vi "Lotis TII LS.vi"() -> ()   [LabVIEW 2015]
doc: "Example VI that demonstrates all library features."
uses:
  PL Lotis TII LS.lvclass
panel:
  in  "baud rate":u32(ring)=57600 items=["4800"=4800, "9600"=9600, "19200"=19200, "38400"=38400, "57600"=57600]
  in  "Tab Control":enum32{"Control", "Information"}(tab)
  in  "stop laser (keep lamp on)":bool
  in  "stop laser":bool
  in  "start laser":bool
  in  "configuration":T1={"device mode"=0, "error code"=0, "number of errors"=0, "cooling system"={"ready"=FALSE, "error"=FALSE}, "lamps"={"frequency, Hz"=0, "channel 1"={"trigger"=1, "state"=1, "energy, J"=0.0}, "channel 2"={"trigger"=1, "state"=1, "energy, J"=0.0}, "amplifier"={"enabled"=FALSE}, "off delay, s"=0, "number of shots"=0, "operation time, min."=0}, "Q-switches"={"frequency, Hz"=0.0, "trigger"=1, "channel 1"={"on"=FALSE, "delay, ns"=0}, "channel 2"={"on"=FALSE, "delay, ns"=0}, "number of shots"=0}, "shutters"={"channel 1"={"open"=FALSE}, "channel 1"={"open"=FALSE}}, "external device state index"=0, "external device flags"=[], "radiation energy, mJ"={"channel 1"=0, "channel 2"=0}, "lamp to Q-switch frequency ratio"=0, "4th harmonic crystal T, °C"=0.0} {"Q-switches"."trigger" items=["always on", "internal", "external (primary)", "external (secondary)", "single shot"]; "lamps"."channel 2"."state" items=["off"=0, "on"=1, "pulses"=3]; "lamps"."channel 2"."trigger" items=["internal"=1, "external"=2, "single shot"=3]; "lamps"."channel 1"."state" items=["off"=0, "on"=1, "pulses"=3]; "lamps"."channel 1"."trigger" items=["internal"=1, "external"=2, "single shot"=3]; "device mode" items=["independent", "primary", "secondary"]}
  in  "reset errors":bool
  out "device name":string
  out "serial number":string
  out "device information":T2 {"optical channels" items=["no", "single", "double", "double with ns delays"]; "cooling system" items=["no", "single", "double", "internal"]; "laser system" items=["single lamp", "double lamp", "long pulse", "double lamp PICO", "single lamp with delay", "extended synchronization"]}
  out "external device states":u8[](array[numeric]) format="%x"
  out "message table index":u8
  out "power supply information":T3
  out "service information":T4
  in  "default":bool
  in  "restore":bool
  in  "save":bool
  in  "port":refnum<visa-resource-name>
  out "error":errorcluster
  in  "stop":bool
  out "Lotis":refnum<class "PL Lotis TII LS.lvclass">
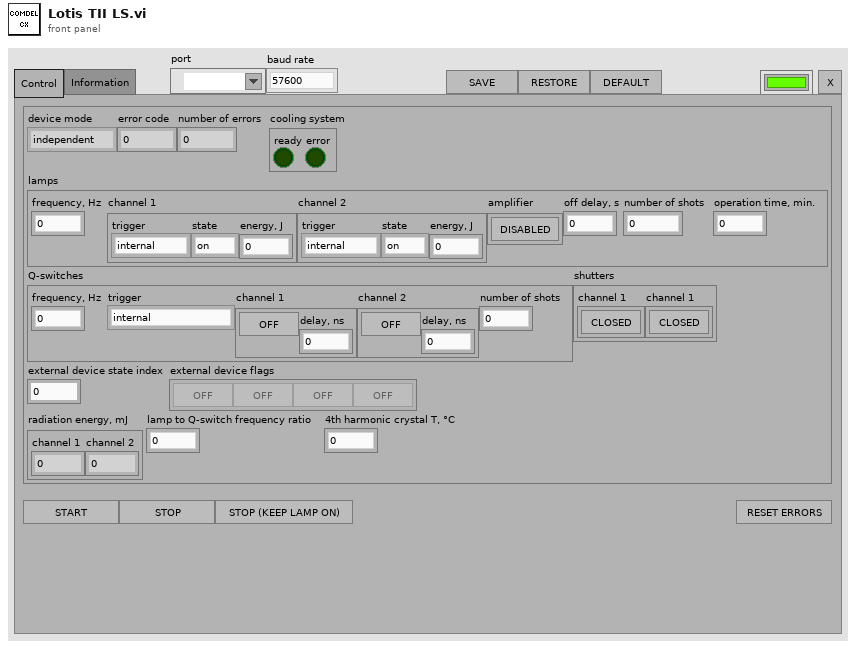
[diagram p1: front panel]
types:
  T1 = cluster{"device mode":u16, "error code":u8, "number of errors":u8, "cooling system":cluster{"ready":bool, "error":bool}, "lamps":cluster{"frequency, Hz":u32, "channel 1":cluster{"trigger":u16, "state":u16, "energy, J":dbl}, "channel 2":cluster{"trigger":u16, "state":u16, "energy, J":dbl}, "amplifier":cluster{"enabled":bool}, "off delay, s":u32, "number of shots":u32, "operation time, min.":u32}, "Q-switches":cluster{"frequency, Hz":dbl, "trigger":u16, "channel 1":cluster{"on":bool, "delay, ns":u32}, "channel 2":cluster{"on":bool, "delay, ns":u32}, "number of shots":u32}, "shutters":cluster{"channel 1":cluster{"open":bool}, "channel 1":cluster{"open":bool}}, "external device state index":u8, "external device flags":bool[], "radiation energy, mJ":cluster{"channel 1":u32, "channel 2":u32}, "lamp to Q-switch frequency ratio":u32, "4th harmonic crystal T, °C":dbl}
  T2 = cluster{"model id":u16, "laser name":string, "laser system":u16, "optical channels":u16, "number of radiation indicators":u16, "cooling system":u16, "control buttons":bool, "external door interlock":bool, "external interlock 1":bool, "external interlock 2":bool, "external lamp control":bool, "saving lamp energy":bool, "variable frequency":bool, "extended frequency range":bool, "FH oven temperature":bool, "external device register":u8, "exernal device flags":bool[], "4th harmonic crystal Tmax, °C":u32, "lamps":cluster{"frequency, Hz":cluster{"min":u32, "max":u32, "default":u32}, "channel 1":cluster{"Emin, J":u32, "Emax, J":u32, "Edefault, J":u32}, "channel 2":cluster{"Emin, J":u32, "Emax, J":u32, "Edefault, J":u32}}, "radiation":cluster{"channel 1":cluster{"Emax, mJ":u32}, "channel 2":cluster{"Emax, mJ":u32}}, "Q-switches":cluster{"channel 1":cluster{"delay step, ns":u32}, "channel 2":cluster{"delay step, ns":u32}}}
  T3 = cluster{"channel 1":cluster{"capacitance, uF":u32, "Urequired, V":u32, "Umeasured, V":u32, "Umin, V":u32, "Umax, V":u32}, "channel 2":cluster{"capacitance, uF":u32, "Urequired, V":u32, "Umeasured, V":u32, "Umin, V":u32, "Umax, V":u32}, "Ucorrection-, V":u32, "Ucorrection+, V":u32, "Udeviation max, %":u32}
  T4 = cluster{"lamp energy averaging":u32, "radiation energy averaging":u32, "lamp shots max":u32, "lamp operaition time  max, min.":u32, "lamp external period min, ms":u32, "lamp external period max, ms":u32}
  T5 = cluster{"device mode":u16, "error code":u8, "number of errors":u8, "cooling system":cluster{"ready":bool, "error":bool}, "lamps":cluster{"frequency, Hz":u32, "channel 1":cluster{"trigger":u16, "state":u16, "energy, J":dbl}, "channel 2":cluster{"trigger":u16, "state":u16, "energy, J":dbl}, "amplifier":cluster{"enabled":bool}, "off delay, s":u32, "number of shots":u32, "operation time, min.":u32}, "Q-switches":cluster{"frequency, Hz":dbl, "trigger":u16, "channel 1":cluster{"on":bool, "delay, ns":u32}, "channel 2":cluster{"on":bool, "delay ,ns":u32}, "number of shots":u32}, "shutters":cluster{"channel 1":cluster{"open":bool}, "channel 2":cluster{"open":bool}}, "external device state index":u8, "exernal device flags":bool[], "radiation energy, mJ":cluster{"channel 1":u32, "channel 2":u32}, "lamp to Q-switch frequency ratio":u32, "4th harmonic crystal T, °C":dbl}
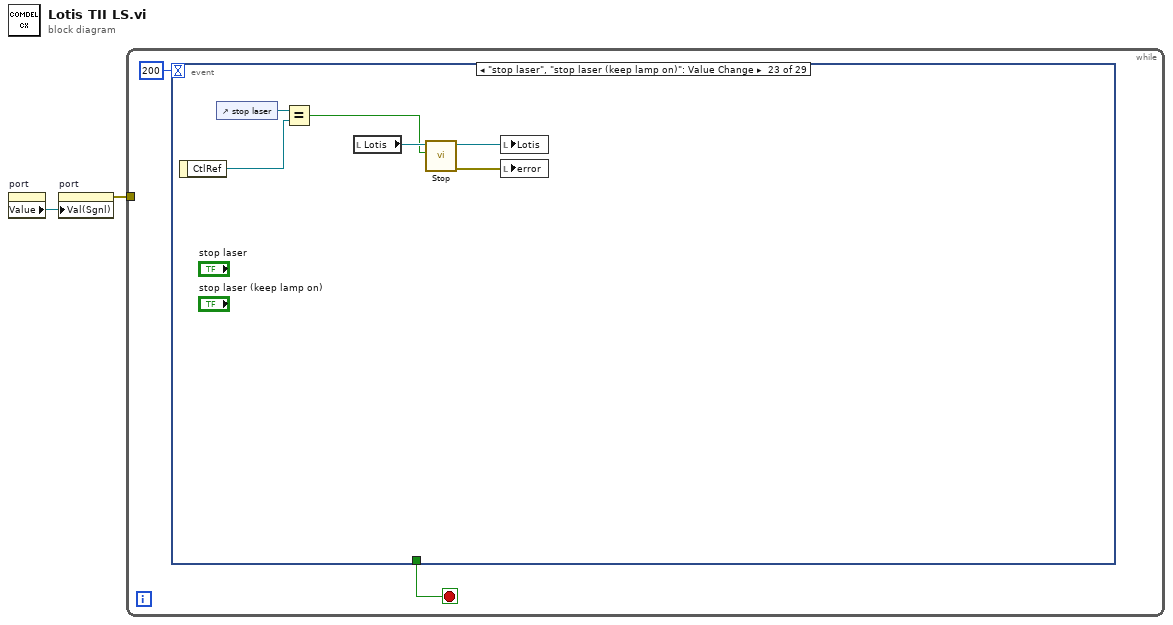
[diagram p0: block diagram]
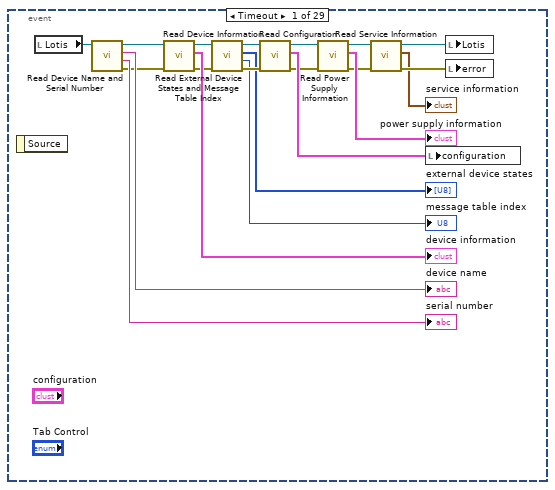
[diagram p2: hidden frame]
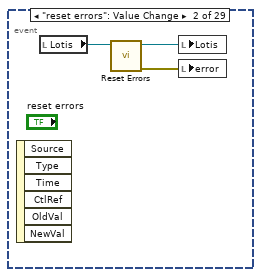
[diagram p3: hidden frame]
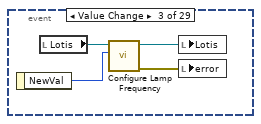
[diagram p4: hidden frame]
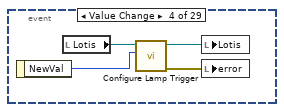
[diagram p5: hidden frame]
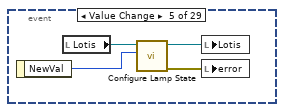
[diagram p6: hidden frame]
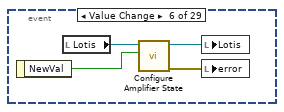
[diagram p7: hidden frame]
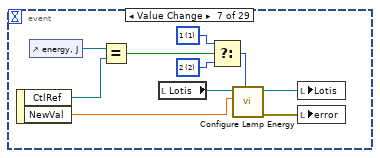
[diagram p8: hidden frame]
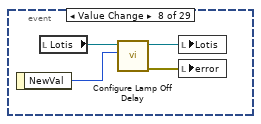
[diagram p9: hidden frame]
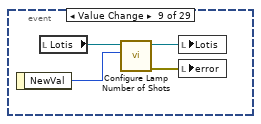
[diagram p10: hidden frame]
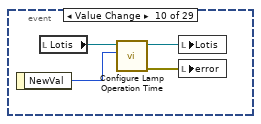
[diagram p11: hidden frame]
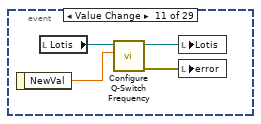
[diagram p12: hidden frame]
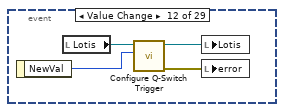
[diagram p13: hidden frame]
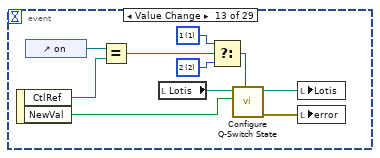
[diagram p14: hidden frame]
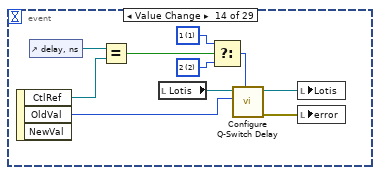
[diagram p15: hidden frame]
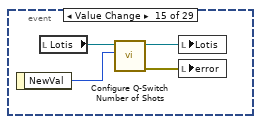
[diagram p16: hidden frame]
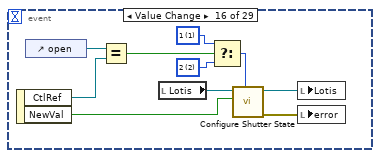
[diagram p17: hidden frame]
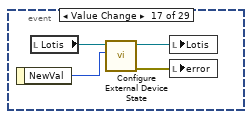
[diagram p18: hidden frame]
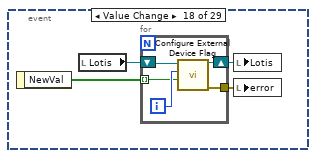
[diagram p19: hidden frame]
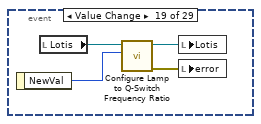
[diagram p20: hidden frame]
diagram:
  n1 = property on="port" class="VISAName"() -> ("Value"=w1:refnum<visa-resource-name>)  [unwired: 2 in, 2 out]
  n2 = property on="port" class="VISAName"("Val(Sgnl)"=w1) -> (error out=w2:errorcluster)  [unwired: 2 in, 1 out]
  n3 = while {
    tunnel: w2 -> [_]
    stop <- w3 stop-if-true
    n4 = event shown="[22] \"stop laser\", \"stop laser (keep lamp on)\": Value Change" {
      selector: _ -> [_ _ _ _ _ _ _ _ _ _ _ _ _ _ _ _ _ _ _ _ _ _ _ _ _ _ _ _ _]
      dyn-events: _ -> [_ _ _ _ _ _ _ _ _ _ _ _ _ _ _ _ _ _ _ _ _ _ _ _ _ _ _ _ _]
      timeout: 200 -> [_ _ _ _ _ _ _ _ _ _ _ _ _ _ _ _ _ _ _ _ _ _ _ _ _ _ _ _ _]
      tunnel: [_ _ _ _ _ _ _ _ _ _ _ _ _ _ _ _ _ _ _ _ _ _ _ _ _ _ _ _ TRUE ("stop")] -> w3
      event Timeout {
        n5 = event-data() -> ()  [unwired: 1 in, 1 out]
        n6 = local read "Lotis"() -> (w25:refnum<class "PL Lotis TII LS.lvclass">)
        n7 = call "Read Device Name and Serial Number.vi"("Lotis in"=w25) -> ("error out"=w21:errorcluster, "serial number"=→"serial number":string, "name"=→"device name":string, "Lotis out"=w22:refnum<class "PL Lotis TII LS.lvclass">)  [unwired: 7 in]
        n8 = call "Read Device Information.vi"("error in (no error)"=w21, "Lotis in"=w22) -> ("error out"=w18:errorcluster, "information"=→"device information":T2, "Lotis out"=w19:refnum<class "PL Lotis TII LS.lvclass">)  [unwired: 7 in]
        n9 = call "Read External Device States and Message Table Index.vi"("error in (no error)"=w18, "Lotis in"=w19) -> ("error out"=w17:errorcluster, "message table index"=→"message table index":u8, "external device states"=→"external device states":u8[], "Lotis out"=w16:refnum<class "PL Lotis TII LS.lvclass">)  [unwired: 6 in]
        n10 = call "Read Configuration.vi"("error in (no error)"=w17, "Lotis in"=w16) -> ("error out"=w11:errorcluster, "configuration"=w13:T5, "Lotis out"=w12:refnum<class "PL Lotis TII LS.lvclass">)  [unwired: 7 in]
        n11 = call "Read Power Supply Information.vi"("error in (no error)"=w11, "Lotis in"=w12) -> ("error out"=w8:errorcluster, "information"=→"power supply information":T3, "Lotis out"=w9:refnum<class "PL Lotis TII LS.lvclass">)  [unwired: 7 in]
        n12 = call "Read Service Information.vi"("error in (no error)"=w8, "Lotis in"=w9) -> ("error out"=w7:errorcluster, "information"=→"service information":T4, "Lotis out"=w6:refnum<class "PL Lotis TII LS.lvclass">)  [unwired: 7 in]
        n13 = local write "configuration"(w13) -> ()
        n14 = local write "Lotis"(w6) -> ()
        n15 = local write "error"(w7) -> ()
      }
      event "reset errors": Value Change {
        n16 = event-data() -> ()  [unwired: 1 in, 6 out]
        n17 = local read "Lotis"() -> (w28:refnum<class "PL Lotis TII LS.lvclass">)
        n18 = call "Reset Errors.vi"("Lotis in"=w28) -> ("error out"=w26:errorcluster, "Lotis out"=w27:refnum<class "PL Lotis TII LS.lvclass">)  [unwired: 9 in]
        n19 = local write "Lotis"(w27) -> ()
        n20 = local write "error"(w26) -> ()
      }
      event "configuration.lamps.frequency, Hz": Value Change {
        n21 = event-data() -> ("NewVal"=w29:u32)  [unwired: 1 in]
        n22 = local read "Lotis"() -> (w30:refnum<class "PL Lotis TII LS.lvclass">)
        n23 = call "Configure Lamp Frequency.vi"("frequency, Hz"=w29, "Lotis in"=w30) -> ("error out"=w31:errorcluster, "Lotis out"=w32:refnum<class "PL Lotis TII LS.lvclass">)  [unwired: 8 in]
        n24 = local write "Lotis"(w32) -> ()
        n25 = local write "error"(w31) -> ()
      }
      event "configuration.lamps.channel 1.trigger": Value Change {
        n26 = event-data() -> ("NewVal"=w33:u16)  [unwired: 1 in]
        n27 = local read "Lotis"() -> (w36:refnum<class "PL Lotis TII LS.lvclass">)
        n28 = call "Configure Lamp Trigger.vi"("trigger"=w33, "Lotis in"=w36) -> ("error out"=w34:errorcluster, "Lotis out"=w35:refnum<class "PL Lotis TII LS.lvclass">)  [unwired: 8 in]
        n29 = local write "Lotis"(w35) -> ()
        n30 = local write "error"(w34) -> ()
      }
      event "configuration.lamps.channel 1.state": Value Change {
        n31 = event-data() -> ("NewVal"=w38:u16)  [unwired: 1 in]
        n32 = local read "Lotis"() -> (w37:refnum<class "PL Lotis TII LS.lvclass">)
        n33 = call "Configure Lamp State.vi"("state"=w38, "Lotis in"=w37) -> ("error out"=w39:errorcluster, "Lotis out"=w40:refnum<class "PL Lotis TII LS.lvclass">)  [unwired: 8 in]
        n34 = local write "Lotis"(w40) -> ()
        n35 = local write "error"(w39) -> ()
      }
      event "configuration.lamps.amplifier.enabled": Value Change {
        n36 = event-data() -> ("NewVal"=w41:bool)  [unwired: 1 in]
        n37 = local read "Lotis"() -> (w44:refnum<class "PL Lotis TII LS.lvclass">)
        n38 = call "Configure Amplifier State.vi"("lamp enabled"=w41, "Lotis in"=w44) -> ("error out"=w42:errorcluster, "Lotis out"=w43:refnum<class "PL Lotis TII LS.lvclass">)  [unwired: 8 in]
        n39 = local write "Lotis"(w43) -> ()
        n40 = local write "error"(w42) -> ()
      }
      event "configuration.lamps.channel 1.energy, J", "configuration.lamps.channel 2.energy, J": Value Change {
        w52 = u16 2 items=["1"=1, "2"=2]
        w51 = u16 1 items=["1"=1, "2"=2]
        n41 = event-data() -> ("CtlRef"=w45:refnum<vi>, "NewVal"=w46:dbl)  [unwired: 1 in]
        n42 = control-ref of="energy, J"() -> (w54:refnum<vi>)
        n43 = Equal?(x=w54, y=w45) -> (x = y?=w53:bool)
        n44 = local read "Lotis"() -> (w50:refnum<class "PL Lotis TII LS.lvclass">)
        n45 = Select(t=w51, s=w53, f=w52) -> (s? t:f=w49:u16)
        n46 = call "Configure Lamp Energy.vi"("channel (1)"=w49, "energy, J"=w46, "Lotis in"=w50) -> ("error out"=w47:errorcluster, "Lotis out"=w48:refnum<class "PL Lotis TII LS.lvclass">)  [unwired: 7 in]
        n47 = local write "Lotis"(w48) -> ()
        n48 = local write "error"(w47) -> ()
      }
      event "configuration.lamps.off delay, s": Value Change {
        n49 = event-data() -> ("NewVal"=w56:u32)  [unwired: 1 in]
        n50 = local read "Lotis"() -> (w55:refnum<class "PL Lotis TII LS.lvclass">)
        n51 = call "Configure Lamp Off Delay.vi"("off delay, s"=w56, "Lotis in"=w55) -> ("error out"=w57:errorcluster, "Lotis out"=w58:refnum<class "PL Lotis TII LS.lvclass">)  [unwired: 8 in]
        n52 = local write "Lotis"(w58) -> ()
        n53 = local write "error"(w57) -> ()
      }
      event "configuration.lamps.number of shots": Value Change {
        n54 = event-data() -> ("NewVal"=w59:u32)  [unwired: 1 in]
        n55 = local read "Lotis"() -> (w60:refnum<class "PL Lotis TII LS.lvclass">)
        n56 = call "Configure Lamp Number of Shots.vi"("number of shots"=w59, "Lotis in"=w60) -> ("error out"=w61:errorcluster, "Lotis out"=w62:refnum<class "PL Lotis TII LS.lvclass">)  [unwired: 8 in]
        n57 = local write "Lotis"(w62) -> ()
        n58 = local write "error"(w61) -> ()
      }
      event "configuration.lamps.operation time, min.": Value Change {
        n59 = event-data() -> ("NewVal"=w63:u32)  [unwired: 1 in]
        n60 = local read "Lotis"() -> (w65:refnum<class "PL Lotis TII LS.lvclass">)
        n61 = call "Configure Lamp Operation Time.vi"("operation time, min."=w63, "Lotis in"=w65) -> ("error out"=w64:errorcluster, "Lotis out"=w66:refnum<class "PL Lotis TII LS.lvclass">)  [unwired: 8 in]
        n62 = local write "Lotis"(w66) -> ()
        n63 = local write "error"(w64) -> ()
      }
      event "configuration.Q-switches.frequency, Hz": Value Change {
        n64 = event-data() -> ("NewVal"=w67:dbl)  [unwired: 1 in]
        n65 = local read "Lotis"() -> (w68:refnum<class "PL Lotis TII LS.lvclass">)
        n66 = call "Configure Q-Switch Frequency.vi"("frequency, Hz"=w67, "Lotis in"=w68) -> ("error out"=w69:errorcluster, "Lotis out"=w70:refnum<class "PL Lotis TII LS.lvclass">)  [unwired: 8 in]
        n67 = local write "Lotis"(w70) -> ()
        n68 = local write "error"(w69) -> ()
      }
      event "configuration.Q-switches.trigger": Value Change {
        n69 = event-data() -> ("NewVal"=w72:u16)  [unwired: 1 in]
        n70 = local read "Lotis"() -> (w71:refnum<class "PL Lotis TII LS.lvclass">)
        n71 = call "Configure Q-Switch Trigger.vi"("trigger"=w72, "Lotis in"=w71) -> ("error out"=w73:errorcluster, "Lotis out"=w74:refnum<class "PL Lotis TII LS.lvclass">)  [unwired: 8 in]
        n72 = local write "Lotis"(w74) -> ()
        n73 = local write "error"(w73) -> ()
      }
      event "configuration.Q-switches.channel 1.on", "configuration.Q-switches.channel 2.on": Value Change {
        w77 = u16 2 items=["1"=1, "2"=2]
        w75 = u16 1 items=["1"=1, "2"=2]
        n74 = event-data() -> ("CtlRef"=w79:refnum<vi>, "NewVal"=w81:bool)  [unwired: 1 in]
        n75 = control-ref of="on"() -> (w80:refnum<vi>)
        n76 = Equal?(x=w80, y=w79) -> (x = y?=w78:bool)
        n77 = local read "Lotis"() -> (w82:refnum<class "PL Lotis TII LS.lvclass">)
        n78 = Select(t=w75, s=w78, f=w77) -> (s? t:f=w76:u16)
        n79 = call "Configure Q-Switch State.vi"("channel (1)"=w76, "on"=w81, "Lotis in"=w82) -> ("error out"=w83:errorcluster, "Lotis out"=w84:refnum<class "PL Lotis TII LS.lvclass">)  [unwired: 7 in]
        n80 = local write "Lotis"(w84) -> ()
        n81 = local write "error"(w83) -> ()
      }
      event "configuration.Q-switches.channel 1.delay, ns", "configuration.Q-switches.channel 2.delay, ns": Value Change {
        w91 = u16 2 items=["1"=1, "2"=2]
        w90 = u16 1 items=["1"=1, "2"=2]
        n82 = event-data() -> ("CtlRef"=w93:refnum<vi>, "OldVal"=w86:u32)  [unwired: 1 in, 1 out]
        n83 = control-ref of="delay, ns"() -> (w94:refnum<vi>)
        n84 = Equal?(x=w94, y=w93) -> (x = y?=w92:bool)
        n85 = local read "Lotis"() -> (w87:refnum<class "PL Lotis TII LS.lvclass">)
        n86 = Select(t=w90, s=w92, f=w91) -> (s? t:f=w88:u16)
        n87 = call "Configure Q-Switch Delay.vi"("channel (1)"=w88, "delay, ns"=w86, "Lotis in"=w87) -> ("error out"=w85:errorcluster, "Lotis out"=w89:refnum<class "PL Lotis TII LS.lvclass">)  [unwired: 7 in]
        n88 = local write "Lotis"(w89) -> ()
        n89 = local write "error"(w85) -> ()
      }
      event "configuration.Q-switches.number of shots": Value Change {
        n90 = event-data() -> ("NewVal"=w95:u32)  [unwired: 1 in]
        n91 = local read "Lotis"() -> (w98:refnum<class "PL Lotis TII LS.lvclass">)
        n92 = call "Configure Q-Switch Number of Shots.vi"("number of shots"=w95, "Lotis in"=w98) -> ("error out"=w96:errorcluster, "Lotis out"=w97:refnum<class "PL Lotis TII LS.lvclass">)  [unwired: 8 in]
        n93 = local write "Lotis"(w97) -> ()
        n94 = local write "error"(w96) -> ()
      }
      event "configuration.shutters.channel 1.open", "configuration.shutters.channel 1.open": Value Change {
        w105 = u16 2 items=["1"=1, "2"=2]
        w104 = u16 1 items=["1"=1, "2"=2]
        n95 = event-data() -> ("CtlRef"=w107:refnum<vi>, "NewVal"=w100:bool)  [unwired: 1 in]
        n96 = control-ref of="open"() -> (w108:refnum<vi>)
        n97 = Equal?(x=w108, y=w107) -> (x = y?=w106:bool)
        n98 = local read "Lotis"() -> (w101:refnum<class "PL Lotis TII LS.lvclass">)
        n99 = Select(t=w104, s=w106, f=w105) -> (s? t:f=w102:u16)
        n100 = call "Configure Shutter State.vi"("channel (1)"=w102, "open"=w100, "Lotis in"=w101) -> ("error out"=w99:errorcluster, "Lotis out"=w103:refnum<class "PL Lotis TII LS.lvclass">)  [unwired: 7 in]
        n101 = local write "Lotis"(w103) -> ()
        n102 = local write "error"(w99) -> ()
      }
      event "configuration.external device state index": Value Change {
        n103 = event-data() -> ("NewVal"=w109:u8)  [unwired: 1 in]
        n104 = local read "Lotis"() -> (w112:refnum<class "PL Lotis TII LS.lvclass">)
        n105 = call "Configure External Device State.vi"("state index"=w109, "Lotis in"=w112) -> ("error out"=w110:errorcluster, "Lotis out"=w111:refnum<class "PL Lotis TII LS.lvclass">)  [unwired: 8 in]
        n106 = local write "Lotis"(w111) -> ()
        n107 = local write "error"(w110) -> ()
      }
      event "configuration.external device flags": Value Change {
        n108 = event-data() -> ("NewVal"=w113:bool[])  [unwired: 1 in]
        n109 = local read "Lotis"() -> (w116:refnum<class "PL Lotis TII LS.lvclass">)
        n110 = for {
          tunnel: [w119] -> w114
          shift-right: [w120] -> w115
          shift-left: w116 -> [w121]
          tunnel: w113 -> [w117] mode=indexing
          i -> [w118]
          n111 = call "Configure External Device Flag.vi"("on"=w117, "flag index"=w118, "Lotis in"=w121) -> ("error out"=w119:errorcluster, "Lotis out"=w120:refnum<class "PL Lotis TII LS.lvclass">)  [unwired: 7 in]
        }
        n112 = local write "Lotis"(w115) -> ()
        n113 = local write "error"(w114) -> ()
      }
      event "configuration.lamp to Q-switch frequency ratio": Value Change {
        n114 = event-data() -> ("NewVal"=w122:u32)  [unwired: 1 in]
        n115 = local read "Lotis"() -> (w123:refnum<class "PL Lotis TII LS.lvclass">)
        n116 = call "Configure Lamp to Q-Switch Frequency Ratio.vi"("ratio"=w122, "Lotis in"=w123) -> ("error out"=w124:errorcluster, "Lotis out"=w125:refnum<class "PL Lotis TII LS.lvclass">)  [unwired: 8 in]
        n117 = local write "Lotis"(w125) -> ()
        n118 = local write "error"(w124) -> ()
      }
      event "configuration.4th harmonic crystal T, °C": Value Change {
        n119 = event-data() -> ("NewVal"=w126:dbl)  [unwired: 1 in]
        n120 = local read "Lotis"() -> (w127:refnum<class "PL Lotis TII LS.lvclass">)
        n121 = call "Configure 4th Harmonic Crystal Temperature.vi"("T, °C"=w126, "Lotis in"=w127) -> ("error out"=w128:errorcluster, "Lotis out"=w129:refnum<class "PL Lotis TII LS.lvclass">)  [unwired: 8 in]
        n122 = local write "Lotis"(w129) -> ()
        n123 = local write "error"(w128) -> ()
      }
      event "save": Value Change {
        n124 = event-data() -> ()  [unwired: 1 in, 1 out]
        n125 = local read "Lotis"() -> (w132:refnum<class "PL Lotis TII LS.lvclass">)
        n126 = call "Save Configuration.vi"("Lotis in"=w132) -> ("error out"=w130:errorcluster, "Lotis out"=w131:refnum<class "PL Lotis TII LS.lvclass">)  [unwired: 9 in]
        n127 = local write "Lotis"(w131) -> ()
        n128 = local write "error"(w130) -> ()
      }
      event "start laser": Value Change {
        n129 = event-data() -> ()  [unwired: 1 in, 1 out]
        n130 = local read "Lotis"() -> (w133:refnum<class "PL Lotis TII LS.lvclass">)
        n131 = call "Start.vi"("Lotis in"=w133) -> ("error out"=w134:errorcluster, "Lotis out"=w135:refnum<class "PL Lotis TII LS.lvclass">)  [unwired: 9 in]
        n132 = local write "Lotis"(w135) -> ()
        n133 = local write "error"(w134) -> ()
      }
      event "stop laser", "stop laser (keep lamp on)": Value Change {
        n134 = event-data() -> ("CtlRef"=w137:refnum<vi>)  [unwired: 1 in]
        n135 = control-ref of="stop laser"() -> (w138:refnum<vi>)
        n136 = Equal?(x=w138, y=w137) -> (x = y?=w136:bool)
        n137 = local read "Lotis"() -> (w139:refnum<class "PL Lotis TII LS.lvclass">)
        n138 = call "Stop.vi"("switch lamp off (true)"=w136, "Lotis in"=w139) -> ("error out"=w140:errorcluster, "Lotis out"=w141:refnum<class "PL Lotis TII LS.lvclass">)  [unwired: 8 in]
        n139 = local write "Lotis"(w141) -> ()
        n140 = local write "error"(w140) -> ()
      }
      event "restore": Value Change {
        n141 = event-data() -> ()  [unwired: 1 in, 1 out]
        n142 = local read "Lotis"() -> (w142:refnum<class "PL Lotis TII LS.lvclass">)
        n143 = call "Restore Configuration.vi"("Lotis in"=w142) -> ("error out"=w143:errorcluster, "Lotis out"=w144:refnum<class "PL Lotis TII LS.lvclass">)  [unwired: 9 in]
        n144 = local write "Lotis"(w144) -> ()
        n145 = local write "error"(w143) -> ()
      }
      event "default": Value Change {
        n146 = event-data() -> ()  [unwired: 1 in, 1 out]
        n147 = local read "Lotis"() -> (w145:refnum<class "PL Lotis TII LS.lvclass">)
        n148 = call "Restore Default Configuration.vi"("Lotis in"=w145) -> ("error out"=w146:errorcluster, "Lotis out"=w147:refnum<class "PL Lotis TII LS.lvclass">)  [unwired: 9 in]
        n149 = local write "Lotis"(w147) -> ()
        n150 = local write "error"(w146) -> ()
      }
      event "port": Value Change {
        n151 = event-data() -> ()  [unwired: 1 in, 6 out]
        n152 = local read "Lotis"() -> (w154:refnum<class "PL Lotis TII LS.lvclass">)
        n153 = call "Close.vi"("Comdel in"=w154) -> ("error out"=w149:errorcluster)  [unwired: 10 in]
        n154 = call <vilib>:"Clear Errors.vi"("error in (no error)"=w149) -> ("error out"=w151:errorcluster)  [unwired: 5 in, 1 out]
        n155 = local read "baud rate"() -> (w148:u32)
        n156 = call "Initialize.vi"("error in (no error)"=w151, "baud rate (57600)"=w148, "port"="port") -> ("error out"=→"error":errorcluster, "Lotis out"=→"Lotis":refnum<class "PL Lotis TII LS.lvclass">)  [unwired: 7 in]
      }
      event "baud rate": Value Change {
        n157 = event-data() -> ("NewVal"=w156:u32)  [unwired: 1 in]
        n158 = local read "Lotis"() -> (w157:refnum<class "PL Lotis TII LS.lvclass">)
        n159 = property on="port" class="VISAName"() -> ("Value"=w155:refnum<visa-resource-name>)  [unwired: 2 in, 2 out]
        n160 = call "Configure Baud Rate.vi"("baud rate"=w156, "Lotis in"=w157) -> ("error out"=w158:errorcluster, "Lotis out"=w159:refnum<class "PL Lotis TII LS.lvclass">)  [unwired: 8 in]
        n161 = property on="port" class="VISAName"("Val(Sgnl)"=w155) -> ()  [unwired: 2 in, 2 out]
        n162 = local write "Lotis"(w159) -> ()
        n163 = local write "error"(w158) -> ()
      }
      event "error": Mouse Up {
        n164 = event-data() -> ()  [unwired: 1 in, 1 out]
        n165 = local read "error"() -> (w160:errorcluster)
        n166 = call <vilib>:"Simple Error Handler.vi"("error in (no error)"=w160) -> ()  [unwired: 4 in, 5 out]
      }
      event "stop": Value Change {
        n167 = event-data() -> ()  [unwired: 1 in, 1 out]
        n168 = local read "Lotis"() -> (w162:refnum<class "PL Lotis TII LS.lvclass">)
        n169 = call "Close.vi"("Comdel in"=w162) -> ("error out"=w161:errorcluster)  [unwired: 10 in]
        n170 = call <vilib>:"Clear Errors.vi"("error in (no error)"=w161) -> ()  [unwired: 5 in, 2 out]
      }
    }
  }
